vi "getSerializedData.vi"(0 "reference":refnum<class "CallEdge.lvclass">, 5 "error in (no error)":errorcluster) -> (14 "reference out":refnum<class "CallEdge.lvclass">, 15 "startNode":refnum<class "AbstractNode.lvclass">, 16 "endNode":refnum<class "AbstractNode.lvclass">, 17 "xmlOut":string, 19 "error out":errorcluster)   [LabVIEW 2012, in "CallEdge.lvclass"]
doc: "getSerializedData"
uses:
  <resource>/Framework/Providers/Open_GDS/UML/CallEdge_class/CallEdge.lvclass
  <resource>/Framework/Providers/Open_GDS/UML/AbstractNode_class/AbstractNode.lvclass
  <resource>/Framework/Providers/Open_GDS/UML/AbstractNode_class/ObjectReference.ctl
  <resource>/Framework/Providers/Open_GDS/UML/LineStyle_class/ObjectReference.ctl
  <resource>/Framework/Providers/Open_GDS/UML/ArrowHead_class/ObjectReference.ctl
  <resource>/Framework/Providers/Open_GDS/UML/General/Point/Point Point2D.ctl
  <resource>/Framework/Providers/Open_GDS/UML/ArrowHead_class/ArrowHead.lvclass
  <resource>/Framework/Providers/Open_GDS/UML/LineStyle_class/LineStyle.lvclass
  <resource>/Framework/Providers/Open_GDS/UML/SegmentedLineEdge_class/SegmentedLineEdge.lvclass
  <resource>/Framework/Providers/Open_GDS/UML/AbstractEdge_class/AbstractEdge.lvclass
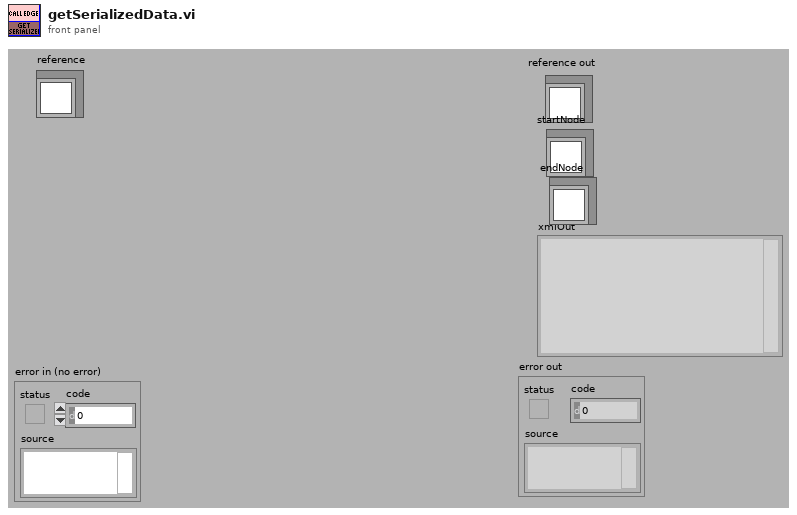
[diagram p1: front panel]
types:
  T1 = typedef "AbstractNode.lvclass/ObjectReference.ctl" = refnum<k1>
  T2 = typedef "LineStyle.lvclass/ObjectReference.ctl" = refnum<k1>
  T3 = typedef "ArrowHead.lvclass/ObjectReference.ctl" = refnum<k1>
  T4 = typedef "Point Point2D.ctl" = cluster{"x":dbl, "y":dbl}
  T5 = cluster{"Base class":cluster{"Base class":cluster{"Base class":cluster{"start":T1, "end":T1}}, "lineStyle":T2, "startArrowHead":T3, "endArrowHead":T3, "startLabel":string, "midLabel":string, "endLabel":string, "MidLabelOffset":T4, "SplitWire":bool}, "signal":bool}
  T6 = typedef "CallEdge.lvclass/ObjectAttributes.ctl" = cluster{"signal":bool}
  T7 = typedef "SegmentedLineEdge.lvclass/ObjectAttributes.ctl" = cluster{"lineStyle":refnum<class "LineStyle.lvclass">, "startArrowHead":refnum<class "ArrowHead.lvclass">, "endArrowHead":refnum<class "ArrowHead.lvclass">, "startLabel":string, "midLabel":string, "endLabel":string, "MidLabelOffset":T4, "SplitWire":bool}
  T8 = typedef "AbstractEdge.lvclass/ObjectAttributes.ctl" = cluster{"start":refnum<class "AbstractNode.lvclass">, "end":refnum<class "AbstractNode.lvclass">}
  T9 = cluster{"Attributes":cluster{"Base class":cluster{"Base class":cluster{"Base class":cluster{"start":T1, "end":T1}}, "lineStyle":T2, "startArrowHead":T3, "endArrowHead":T3, "startLabel":string, "midLabel":string, "endLabel":string, "MidLabelOffset":T4, "SplitWire":bool}, "signal":bool}, "Type(String)":string, "Object name":string, "Object name":string}
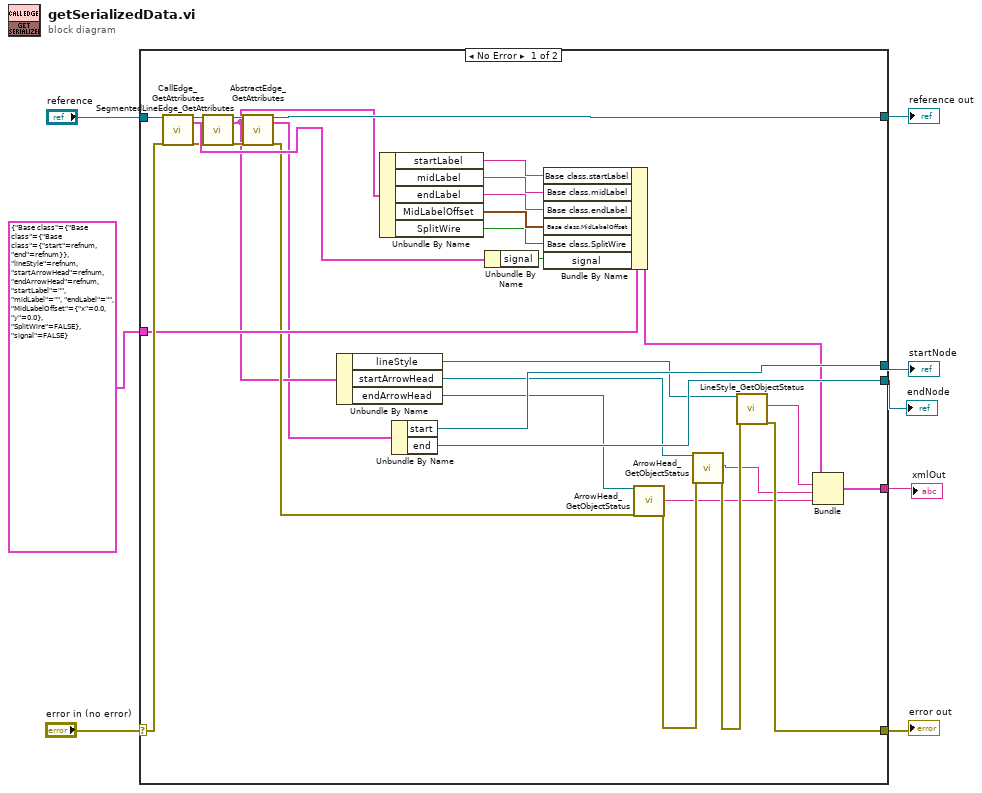
[diagram p0: block diagram]
diagram:
  n1 = case shown="No Error" "error in (no error)" {
    selector: "error in (no error)" -> [w40 w41]
    tunnel: "reference" -> [w39 w42]
    tunnel: [w29 w41] -> w6
    tunnel: [w14 w42] -> w5
    tunnel: [w37 _] -> w4
    tunnel: [w36 _] -> w3
    tunnel: [w35 _] -> w2
    tunnel: T5 {"Base class"={"Base class"={"Base class"={"start"=refnum, "end"=refnum}}, "lineStyle"=refnum, "startArrowHead"=refnum, "endArrowHead"=refnum, "startLabel"="", "midLabel"="", "endLabel"="", "MidLabelOffset"={"x"=0.0, "y"=0.0}, "SplitWire"=FALSE}, "signal"=FALSE} ("Attributes") -> [w28 _]
    frame No Error {
      n2 = call <resource>:"CallEdge_GetAttributes.vi"("reference in"=w39, "error in (no error)"=w40) -> ("reference out"=w19:refnum<class "CallEdge.lvclass">, "Data"=w20:T6, "error out"=w18:errorcluster)  [unwired: 1 in, 14 out]
      n3 = call <resource>:"SegmentedLineEdge_GetAttributes.vi"("reference in"=w19, "error in (no error)"=w18) -> ("reference out"=w17:refnum<class "CallEdge.lvclass">, "Data"=w13:T7, "error out"=w16:errorcluster)  [unwired: 14 in, 1 out]
      n4 = call <resource>:"AbstractEdge_GetAttributes.vi"("reference in"=w17, "error in (no error)"=w16) -> ("reference out"=w14:refnum<class "CallEdge.lvclass">, "Data"=w12:T8, "error out"=w15:errorcluster)  [unwired: 14 in, 1 out]
      n5 = Unbundle By Name(w13) -> ("lineStyle"=w34:refnum<class "LineStyle.lvclass">, "startArrowHead"=w33:refnum<class "ArrowHead.lvclass">, "endArrowHead"=w32:refnum<class "ArrowHead.lvclass">)
      n6 = Unbundle By Name(w13) -> ("startLabel"=w27:string, "midLabel"=w26:string, "endLabel"=w25:string, "MidLabelOffset"=w24:T4, "SplitWire"=w23:bool)
      n7 = Unbundle By Name(w12) -> ("start"=w36:refnum<class "AbstractNode.lvclass">, "end"=w35:refnum<class "AbstractNode.lvclass">)
      n8 = Unbundle By Name(w20) -> ("signal"=w22:bool)
      n9 = Bundle By Name(cluster=w28, "Base class.startLabel"=w27, "Base class.midLabel"=w26, "Base class.endLabel"=w25, "Base class.MidLabelOffset"=w24, "Base class.SplitWire"=w23, "signal"=w22) -> (w21:T5)
      n10 = call <resource>:"ArrowHead_GetObjectStatus.vi"("reference in"=w32, "error in (no error)"=w15) -> ("Object name"=w9:string, "error out"=w31:errorcluster)  [unwired: 1 in, 15 out]
      n11 = call <resource>:"ArrowHead_GetObjectStatus.vi"("reference in"=w33, "error in (no error)"=w31) -> ("Object name"=w10:string, "error out"=w30:errorcluster)  [unwired: 1 in, 15 out]
      n12 = call <resource>:"LineStyle_GetObjectStatus.vi"("reference"=w34, "error in (no error)"=w30) -> ("Type(String)"=w11:string, "error out"=w29:errorcluster)  [unwired: 15 in, 1 out]
      n13 = Bundle("Attributes"=w21, "Type(String)"=w11, "Object name"=w10, "Object name"=w9) -> (w38:T9)  [unwired: 1 out]
      n14 = Flatten To XML(anything=w38) -> (xml string=w37:string)
    }
    frame Error {
    }
  }
  "reference out" <- w5
  "error out" <- w6
  "startNode" <- w3
  "endNode" <- w2
  "xmlOut" <- w4
